vi "Motic Activate Cooler.vi"(8 "error in (no error)":errorcluster, 10 "activate":bool, 11 "camera":i32) -> (0 "error out":errorcluster, 2 "activation result":bool, 3 "camera out":i32)   [LabVIEW 2012, in "MoticApi.lvlib"]
doc: "MOTICAPI bool Motic_ActivateCooler(MUCam_Handle camera, bool act);"
uses:
  MoticApi.lvlib
  MoticApi.dll
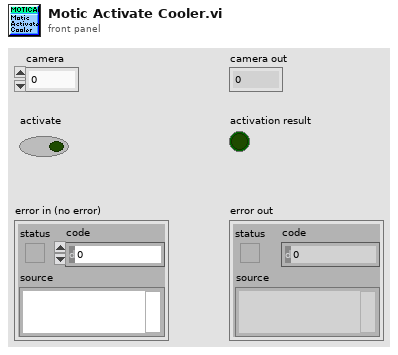
[diagram p1: front panel]
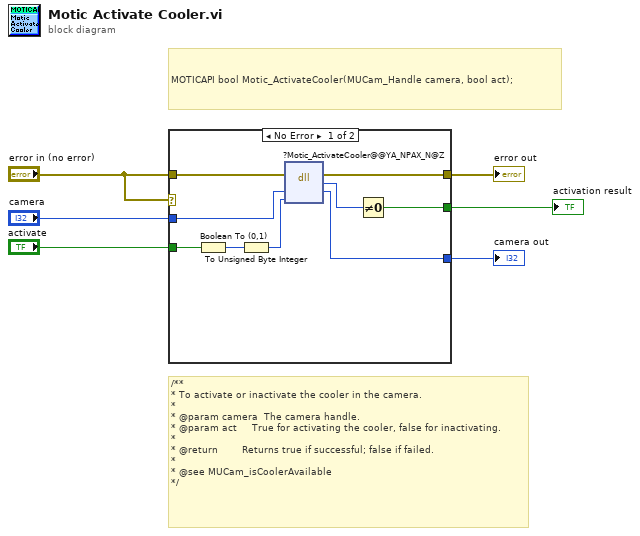
[diagram p0: block diagram]
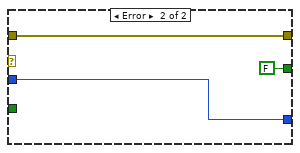
[diagram p2: hidden frame]
diagram:
  # "/**\n* To activate or inactivate the cooler in the camera.\n*\n* @param camera  The camera handle.\n* @param act     True for activating the cooler, false for inactivating.\n*\n* @return        Returns true if successful; false if failed.\n*\n* @see MUCam_isCoolerAvailable\n*/"
  # "MOTICAPI bool Motic_ActivateCooler(MUCam_Handle camera, bool act);"
  n1 = case shown="No Error" "error in (no error)" {
    tunnel: [w15 FALSE] -> w6
    tunnel: "camera" -> [w13 w16]
    tunnel: [w12 w16] -> w4
    tunnel: "activate" -> [w11 _]
    tunnel: "error in (no error)" -> [w10 w18]
    tunnel: [w9 w18] -> w2
    frame No Error {
      n2 = Boolean To (0,1)(Boolean=w11) -> (0, 1=w8:i16)
      n3 = To Unsigned Byte Integer(number=w8) -> (unsigned 8bit integer=w7:u8)
      n4 = dll-call lib="C:/Users/TTS-Digital/Desktop/MoticApi/MoticApi_git/MoticApi/MoticApi.*" fn="?Motic_ActivateCooler@@YA_NPAX_N@Z"(error in=w10, "camera"=w13, "activate"=w7) -> (error out=w9:errorcluster, w14:u8, "camera"=w12:i32)  [unwired: 3 in, 1 out]
      n5 = Not Equal To 0?(x=w14) -> (x != 0?=w15:bool)
    }
    frame Error {
    }
  }
  "activation result" <- w6
  "camera out" <- w4
  "error out" <- w2
